vi "Test OpenCVFaceDetect.vi"() -> ()   [LabVIEW 2021]
uses:
  OpenCVCam/OpenCVCam.lvclass
  OpenCVFaceDetection.lvclass
  .Externals/Library_UserInterface_FrontPanelControl/FrontPanelControl/FrontPanelControl.lvclass
  C:/Localdata/Projects/TriekselSoft/TriekselsoftApplicationFramework/Source/.Externals/Library_YAF/YAFTAF/YAFTAF.lvclass
  C:/Localdata/Projects/TriekselSoft/TriekselsoftApplicationFramework/Source/.Externals/Library_YAF/YActor/YActor.lvclass
  C:/Localdata/Projects/TriekselSoft/TriekselsoftApplicationFramework/Source/.Externals/Interface_UserInterface_IFrontPanel/IFrontPanel/IFrontPanel.lvclass
  C:/Localdata/Projects/TriekselSoft/TriekselsoftApplicationFramework/Source/IInterface/IInterface.lvclass
  C:/Localdata/Projects/TriekselSoft/TriekselsoftApplicationFramework/Source/.Externals/Interface_Object_ICreateDestroy/ICreateDestroy/ICreateDestroy.lvclass
  C:/Localdata/Projects/TriekselSoft/TriekselsoftApplicationFramework/Source/.Externals/Interface_Object_IPersistentData/IPersistentData/IPersistentData.lvclass
  C:/Localdata/Projects/TriekselSoft/TriekselsoftApplicationFramework/Source/.Externals/Interface_TAF_ITAFObject/ITAFObject/ITAFObject.lvclass
  C:/Localdata/Projects/TriekselSoft/TriekselsoftApplicationFramework/Source/YAFTAFObjects/OpenCVFaceDetection/OpenCVFaceDetection.lvclass
  C:/Localdata/Projects/TriekselSoft/TriekselsoftApplicationFramework/Source/.Externals/INewOpenCVMat/INewOpenCVMat.lvclass
panel:
  in  "stop":bool
  out "2D Picture":picture
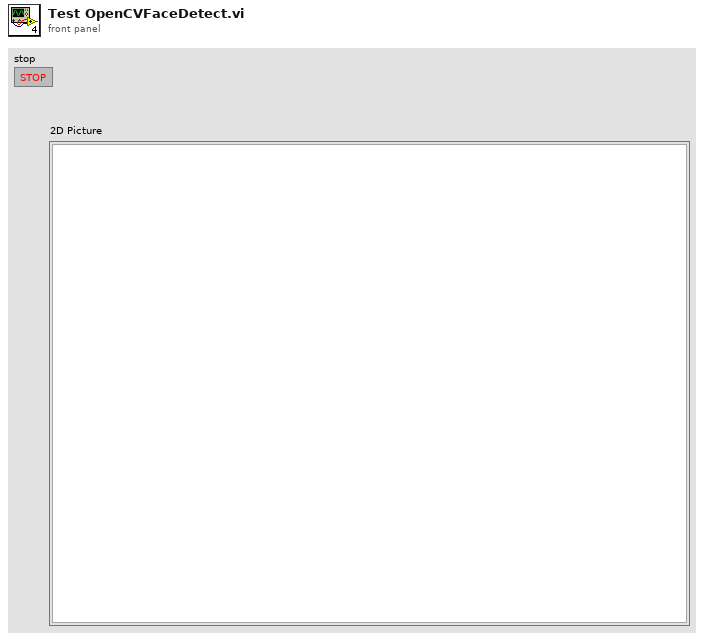
[diagram p1: front panel]
types:
  T1 = typedef "ClusterArrayConversion.lvlib/BundledArray.ctl" = cluster{"Label":string, "Object":refnum<class>, "Array":bool}
  T2 = typedef "imagedata.ctl" = cluster{"image type":i32, "image depth":i32, "image":u8[], "mask":u8[], "colors":u32[], "Rectangle":cluster{"left":i16, "top":i16, "right":i16, "bottom":i16}}
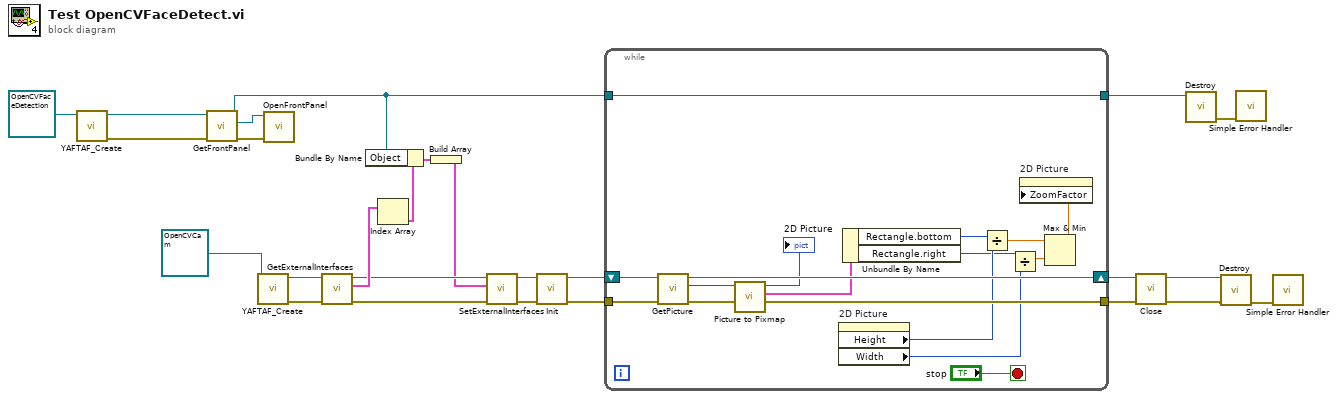
[diagram p0: block diagram]
diagram:
  n1 = call-dynamic "YAFTAF_Create.vi"("object in"=refnum<class "OpenCVFaceDetection.lvclass"> refnum ("OpenCVFaceDetection")) -> ("Error Out"=w6:errorcluster, "object out"=w7:refnum<class "OpenCVFaceDetection.lvclass">)  [unwired: 9 in]
  n2 = call-dynamic "GetFrontPanel.vi"("Error In"=w6, "object in"=w7) -> ("Error Out"=w5:errorcluster, "FrontPanelControl"=w4:refnum<class "FrontPanelControl.lvclass">, "object out"=w3:refnum<class "OpenCVFaceDetection.lvclass">)  [unwired: 7 in]
  n3 = call-dynamic "YAFTAF_Create.vi"("object in"=refnum<class "OpenCVCam.lvclass"> refnum ("OpenCVCam")) -> ("Error Out"=w16:errorcluster, "object out"=w17:refnum<class "OpenCVCam.lvclass">)  [unwired: 9 in]
  n4 = call-dynamic "OpenFrontPanel.vi"("Error In"=w5, "object in"=w4) -> ()  [unwired: 8 in, 2 out]
  n5 = call-dynamic "GetExternalInterfaces.vi"("Error In"=w16, "object in"=w17) -> ("Error Out"=w15:errorcluster, "ExternalInterfaces"=w14:T1[], "object out"=w11:refnum<class "OpenCVCam.lvclass">)  [unwired: 7 in]
  n6 = Index Array(array=w14) -> (element=w13:T1)  [unwired: 1 in]
  n7 = Bundle By Name(cluster=w13, "Object"=w3) -> (w9:T1)
  n8 = Build Array(w9) -> (w8:T1[])
  n9 = call-dynamic "SetExternalInterfaces.vi"("Error In"=w15, "ExternalInterfaces"=w8, "object in"=w11) -> ("Error Out"=w12:errorcluster, "object out"=w10:refnum<class "OpenCVCam.lvclass">)  [unwired: 7 in]
  n10 = call-dynamic "Init.vi"("error in (no error)"=w12, "OpenCVCam in"=w10) -> ("error out"=w25:errorcluster, "OpenCVCam out"=w26:refnum<class "OpenCVCam.lvclass">)  [unwired: 8 in]
  n11 = while {
    shift-right: [w39] -> w23
    shift-left: w26 -> [w42]
    tunnel: w25 -> [w41]
    tunnel: [w40] -> w24
    tunnel: [w27] -> w2
    tunnel: w3 -> [w27]
    stop <- "stop" stop-if-true
    n12 = call-dynamic "GetPicture.vi"("error in (no error)"=w41, "OpenCVCam in"=w42) -> ("error out"=w40:errorcluster, "2D Picture"=w37:picture, "OpenCVCam out"=w39:refnum<class "OpenCVCam.lvclass">)  [unwired: 7 in]
    n13 = call <vilib>:"Picture to Pixmap.vi"("picture"=w37) -> ("image data"=w35:T2, "new picture"=→"2D Picture":picture)  [unwired: 9 in]
    n14 = property on="2D Picture" class="Pict"() -> ("Height"=w33:u32, "Width"=w31:u32)  [unwired: 2 in, 2 out]
    n15 = Unbundle By Name(w35) -> ("Rectangle.bottom"=w34:i16, "Rectangle.right"=w32:i16)
    n16 = Divide(x=w34, y=w33) -> (x/y=w29:dbl)
    n17 = Divide(x=w32, y=w31) -> (x/y=w30:dbl)
    n18 = Max & Min(x=w29, y=w30) -> (max(x,y)=w28:dbl)  [unwired: 1 out]
    n19 = property on="2D Picture" class="Pict"("ZoomFactor"=w28) -> ()  [unwired: 2 in, 2 out]
  }
  n20 = call-dynamic "Close.vi"("error in (no error)"=w24, "OpenCVCam in"=w23) -> ("error out"=w21:errorcluster, "OpenCVCam out"=w22:refnum<class "OpenCVCam.lvclass">)  [unwired: 8 in]
  n21 = call-dynamic "Destroy.vi"("object in"=w2) -> ("Error Out"=w1:errorcluster)  [unwired: 9 in, 1 out]
  n22 = call-dynamic "Destroy.vi"("Error In"=w21, "object in"=w22) -> ("Error Out"=w20:errorcluster)  [unwired: 8 in, 1 out]
  n23 = call <vilib>:"Simple Error Handler.vi"("error in (no error)"=w1) -> ()  [unwired: 4 in, 5 out]
  n24 = call <vilib>:"Simple Error Handler.vi"("error in (no error)"=w20) -> ()  [unwired: 4 in, 5 out]
